vi "Intra-Move Items.vi"(4 "indent":i32, 6 "Insertion index":i32, 8 "error in (no error)":errorcluster, 9 "Copy?":bool, 10 "Indices to move":i32[](array[numeric]), 11 "BetterHandle in":refnum<class "BetterHandle.lvclass">) -> (0 "error out":errorcluster, 3 "BetterHandle out":refnum<class "BetterHandle.lvclass">)   [LabVIEW 2020, in "BetterDragAndDrop.lvlib" / "BetterHandle.lvclass"]
uses:
  BetterHandle.lvclass
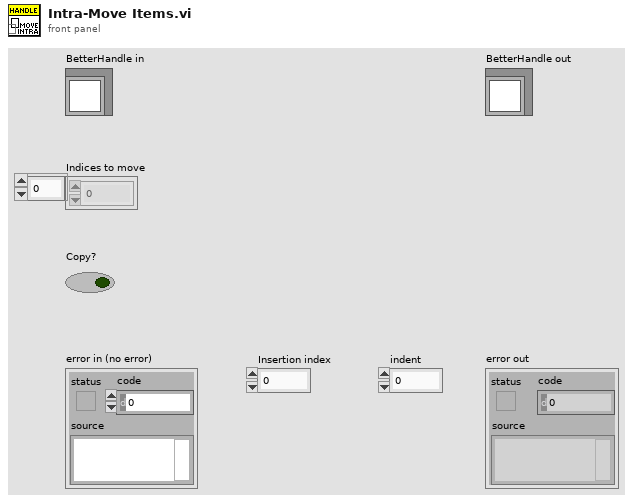
[diagram p1: front panel]
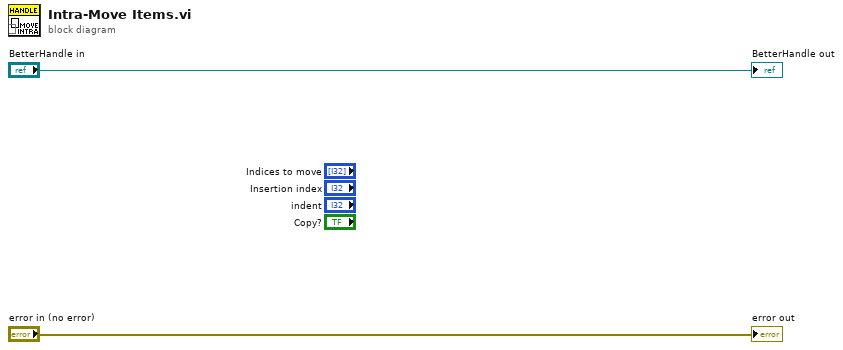
[diagram p0: block diagram]
diagram:
  "error out" <- "error in (no error)"
  "BetterHandle out" <- "BetterHandle in"
